vi "Destroy.vi"(0 "reference in":refnum<class "SlideFeedCommand.lvclass">, 5 "error in (no error)":errorcluster) -> (14 "reference out":refnum<class "SlideFeedCommand.lvclass">, 19 "error out":errorcluster)   [LabVIEW 2013, in "SlideFeedCommand.lvclass"]
doc: "Destructor."
uses:
  SlideFeedCommand.lvclass
  Command_class/Command.lvclass
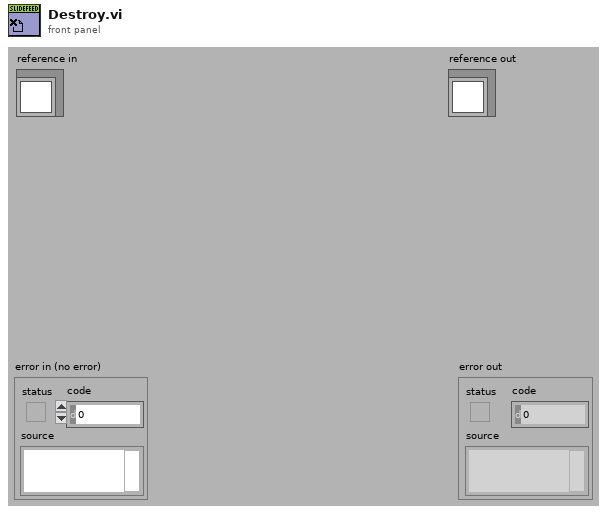
[diagram p1: front panel]
types:
  T1 = typedef "SlideFeedCommand.lvclass/ObjectAttributes.ctl" = cluster{"Slide.lvclass":refnum<class "Slide.lvclass">}
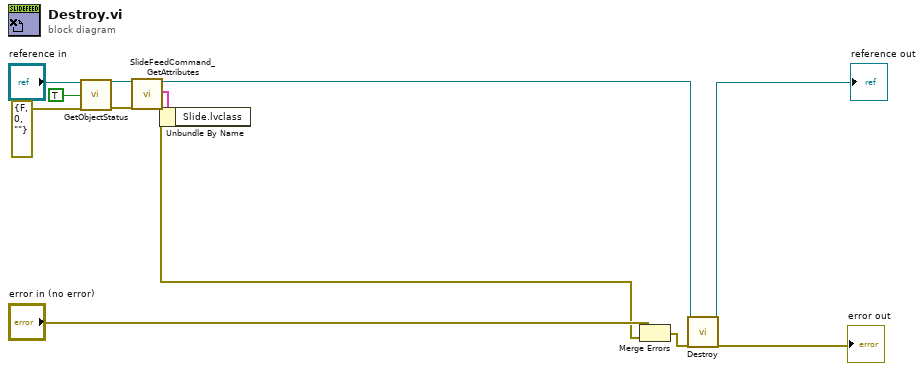
[diagram p0: block diagram]
diagram:
  n1 = call-dynamic "GetObjectStatus.vi"("reference in"="reference in", "simple info (F)"=TRUE ("simple info"), "error in (no error)"=errorcluster {"status"=FALSE, "code"=0, "source"=""}) -> ("reference out"=w5:refnum<class "SlideFeedCommand.lvclass">, "error out"=w6:errorcluster)  [unwired: 5 in, 10 out]
  n2 = call "SlideFeedCommand_GetAttributes.vi"("reference in"=w5, "error in (no error)"=w6) -> ("reference out"=w4:refnum<class "SlideFeedCommand.lvclass">, "attributes"=w3:T1, "error out"=w7:errorcluster)  [unwired: 14 in, 1 out]
  n3 = Unbundle By Name(w3) -> ()  [unwired: 1 out]
  n4 = Merge Errors("error in (no error)", w7) -> (w11:errorcluster)
  n5 = call-parent "Destroy.vi"("reference in"=w4, "error in (no error)"=w11) -> ("reference out"=→"reference out":refnum<class "SlideFeedCommand.lvclass">, "error out"=→"error out":errorcluster)  [unwired: 16 in]
